vi "Launcher.vi"() -> ()   [LabVIEW 2015]
uses:
  ModbusOverMOXA.lvlib
panel:
  in  "String":string
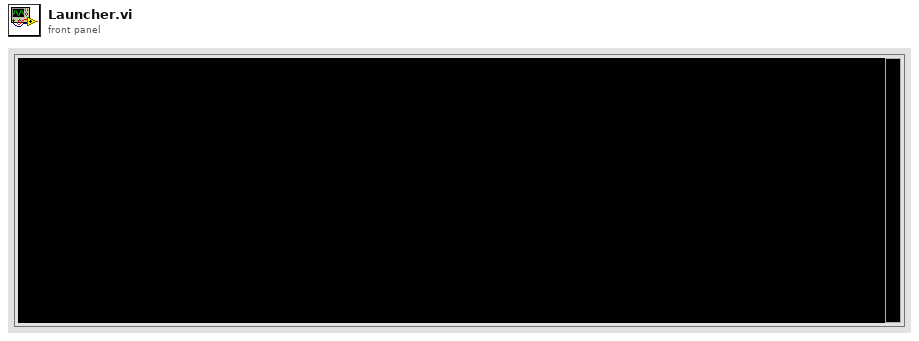
[diagram p1: front panel]
types:
  T1 = cluster{"MQTT":string, "Serializer":string, "Messages":string}
  T2 = typedef "ModbusOverMOXA.lvlib/Broadcast Events--cluster.ctl" = cluster{"Module Did Init":refnum<user-event>, "Status Updated":refnum<user-event>, "Error Reported":refnum<user-event>, "Module Did Stop":refnum<user-event>, "Update Module Execution Status":refnum<user-event>}
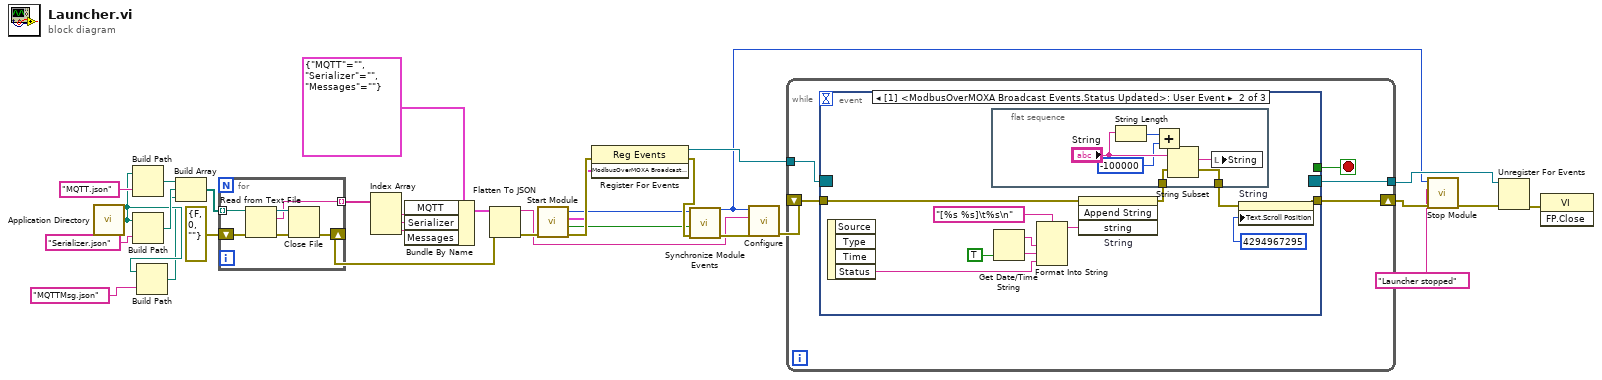
[diagram p0: block diagram]
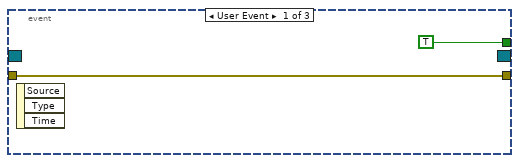
[diagram p2: hidden frame]
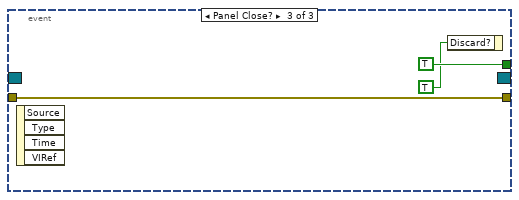
[diagram p3: hidden frame]
diagram:
  n1 = call <vilib>:"Application Directory.vi"() -> ("Application Directory"=w20:path)
  n2 = Build Path(base path=w20, name or relative path="MQTT.json") -> (appended path=w31:path)
  n3 = Build Path(base path=w20, name or relative path="Serializer.json") -> (appended path=w32:path)
  n4 = Build Path(base path=w20, name or relative path="MQTTMsg.json") -> (appended path=w18:path)
  n5 = Build Array(w31, w32, w18) -> (w30:path[])
  n6 = for {
    tunnel: w30 -> [w35] mode=indexing
    tunnel: [w36] -> w28 mode=indexing
    shift-right: [w34] -> w21
    shift-left: errorcluster {"status"=FALSE, "code"=0, "source"=""} ("error out") -> [w33]
    n7 = Read from Text File(file (use dialog)=w35, error in=w33) -> (refnum out=w37:refnum<file>, text=w36:string, error out=w38:errorcluster)  [unwired: 2 in, 1 out]
    n8 = Close File(refnum=w37, error in=w38) -> (error out=w34:errorcluster)  [unwired: 1 out]
  }
  n9 = Index Array(array=w28) -> (element #1=w24:string, element #2=w23:string, element #3=w17:string)  [unwired: 3 in]
  n10 = Bundle By Name(cluster=T1 {"MQTT"="", "Serializer"="", "Messages"=""}, "MQTT"=w24, "Serializer"=w23, "Messages"=w17) -> (w22:T1)
  n11 = Flatten To JSON(anything=w22, error in (no error)=w21) -> (JSON string=w8:string, 11:w16:errorcluster)  [unwired: 1 in]
  n12 = call "Start Module.vi"("error in (no error)"=w16) -> ("error out"=w15:errorcluster, "Wait for Event Sync?"=w11:bool, "ModbusOverMOXA Broadcast Events"=w14:T2, "Module ID"=w12:i32)  [unwired: 7 in]
  n13 = register-events(error in=w15, w14) -> (reference out=w10:refnum<event-registration>, error out=w13:errorcluster)  [unwired: 1 in]
  n14 = call "Synchronize Module Events.vi"("error in (no error)"=w13, "Wait for Event Sync?"=w11, "Module ID"=w12) -> ("error out"=w9:errorcluster, "Module ID (dup)"=w2:i32)  [unwired: 7 in]
  n15 = call "Configure.vi"("error in (no error)"=w9, "Jsonconfig"=w8, "Module ID"=w2) -> ("error out"=w7:errorcluster)  [unwired: 8 in]
  n16 = while {
    tunnel: w10 -> [w43]
    shift-right: [w42] -> w6
    shift-left: w7 -> [w41]
    tunnel: [w40] -> w3
    stop <- w39 stop-if-true
    n17 = event shown="[1] <ModbusOverMOXA Broadcast Events.Status Updated>: User Event" {
      selector: w43 -> [_ _ _]
      dyn-events: [_ _ _] -> w40
      timeout: _ -> [_ _ _]
      tunnel: [w45 w49 w63] -> w42
      tunnel: w41 -> [w45 w56 w63]
      tunnel: [TRUE _ TRUE] -> w39
      event User Event {
        n18 = event-data() -> ()  [unwired: 1 in, 3 out]
      }
      event User Event {
        n19 = event-data() -> ("Status"=w51:string)  [unwired: 1 in, 3 out]
        n20 = flat-sequence {
          tunnel: [w62] -> w47
          tunnel: w46 -> [w62]
          frame #0 {
            n21 = String Length(string="String") -> (length=w59:i32)
            n22 = Add(x=w59, y=-100000 ("offset (0)")) -> (x+y=w57:i32)
            n23 = String Subset(string="String", offset (0)=w57) -> (substring=w61:string)  [unwired: 1 in]
            n24 = local write "String"(w61) -> ()
          }
        }
        n25 = Get Date/Time String(want seconds? (F)=TRUE) -> (date string=w53:string, time string=w52:string)  [unwired: 2 in]
        n26 = Format Into String(format string="[%s %s]\t%s\n", w53, w52, w51) -> (resulting string=w50:string)  [unwired: 2 in, 1 out]
        n27 = invoke on="String" class="Str" method="Append String"(error in=w56, "string"=w50) -> (error out=w46:errorcluster)  [unwired: 2 in, 3 out]
        n28 = property on="String" class="Str"(error in=w47, "Text.Scroll Position"=u32 4294967295) -> (error out=w49:errorcluster)  [unwired: 1 in, 1 out]
      }
      event Panel Close? {
        n29 = event-data() -> ()  [unwired: 1 in, 4 out]
        n30 = event-data("Discard?"=TRUE) -> ()  [unwired: 1 in, 1 out]
      }
    }
  }
  n31 = call "Stop Module.vi"("error in (no error)"=w6, "Origin"="Launcher stopped", "Module ID"=w2) -> ("error out"=w4:errorcluster)  [unwired: 8 in]
  n32 = Unregister For Events(event registration refnum=w3, error in=w4) -> (error out=w5:errorcluster)
  n33 = invoke class="VI" method="FP.Close"(error in=w5) -> ()  [unwired: 2 in, 3 out]
